vi "Main.vi"() -> ()   [LabVIEW 2010]
uses:
  <vilib>/Platform/storage/lvStorage.llb/xStorage/Open Data Storage/Open Data Storage.xnode
  <vilib>/Platform/storage/lvStorage.llb/xStorage/Set Properties/Set Properties.xnode
  <vilib>/Platform/storage/lvStorage.llb/xStorage/Write Data/Write Data.xnode
  <vilib>/Platform/storage/Storage.llb/usiOverwriteOptions.ctl
  <vilib>/Platform/storage/Storage.llb/usiSequenceRepresentation.ctl
  <vilib>/Platform/storage/lvStorage.llb/xStorage/Close Data Storage/Close Data Storage.xnode
  <instrlib>/Tektronix DPO MSO 2000 4000 Series/Public/Data/Read (Single Waveform).vi
  <instrlib>/Tektronix DPO MSO 2000 4000 Series/Public/Data/Read (Multiple Waveforms).vi
  <instrlib>/Tektronix DPO MSO 2000 4000 Series/Public/Configure/Configure Math (Dual).vi
  <vilib>/Platform/storage/lvStorage.llb/_openStorageWithRootAutoDetect.vi
  <vilib>/Platform/storage/lvStorage.llb/xStorage/xStorageSupp/ErrorOut.vi
  <vilib>/Platform/storage/Storage.llb/__savePropString.vi
  <vilib>/Platform/storage/Storage.llb/__savePropTime.vi
  <vilib>/Platform/storage/Storage.llb/_createExplicitChildObject.vi
  <vilib>/Platform/storage/lvStorage.llb/_prepDDT.vi
  <vilib>/Platform/storage/lvStorage.llb/_getChannelNameFromDDT.vi
  <vilib>/Platform/storage/lvStorage.llb/_saveDDT.vi
  <vilib>/Platform/storage/Storage.llb/Get Object Info.vi
  <vilib>/Platform/storage/Storage.llb/__closeStorageFromObject.vi
  <instrlib>/Tektronix DPO MSO 2000 4000 Series/Tektronix DPO MSO 2000 4000 Series.lvlib
panel:
  out "concatenated string":string
  out "Path 3":path
  out "error out":errorcluster
  out "down":bool
  out "up":bool
  out "DOWN":dbl
  out "UP":dbl
  in  "Error Range":dbl min=0.0 max=5.0 step=0.1 format="%#.3g"
  in  "Port to test":u16(ring) items=["AMB 1", "AMB 2", "AMB 3", "AMB 4", "AMB 5", "AMB 18"]
  in  "Assembled by":string="Alexis Ibarra"
  in  "ABM-S/N":string
  in  "IP Addres":string
  in  "Tab Control":T1(tab)
  in  "Start TEST":bool
  out "TIMA":waveform(dbl)(graph)
  out "TIMB":waveform(dbl)(graph)
  out "Differential Signal":waveform(dbl)(graph)
  out "TE Signals":waveform(dbl)[](graph)
  in  "Maximum Time (10000ms)":u32=20000
  in  "Channel B (1: Channel 2)":u16(ring)=1 items=["Channel 1", "Channel 2", "Channel 3", "Channel 4", "Math", "Reference 1", "Reference 2", "Reference 3", "Reference 4"]
  in  "Channel A (0: Channel 1)":u16(ring) items=["Channel 1", "Channel 2", "Channel 3", "Channel 4", "Math", "Reference 1", "Reference 2", "Reference 3", "Reference 4"]
  out "Periode":dbl
  out "Averenge":dbl
  out "STATUS":string
  # "ABM Verification System"
  # "%"
  # "Copyrigth Alexis Ibarrra A. ALMA  Computing"
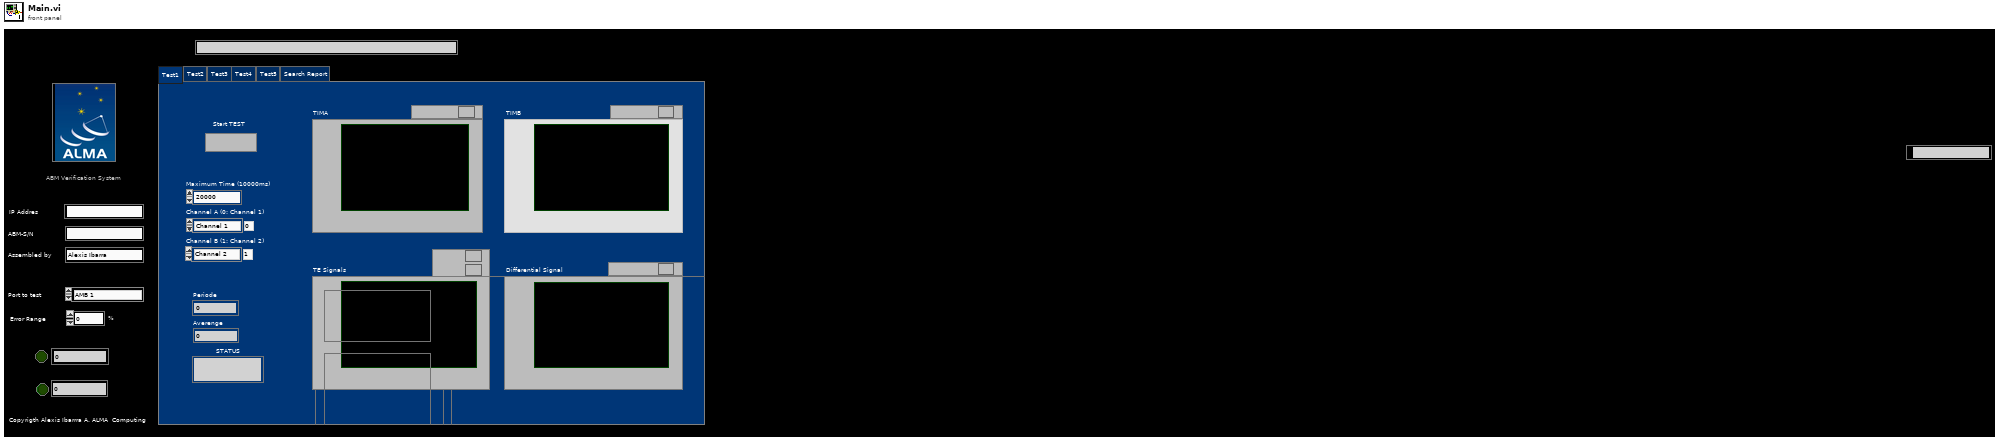
[diagram p1: front panel]
types:
  T1 = enum32{"Test1", "Test2", "Test3", "Test4", "Test5", "Search Report"}
  T2 = enum16{"open", "open or create", "create or replace", "create", "open (read only)"}
  T3 = enum16{"UPDATE", "READ", "QUERY", "CREATE CHILD", "CREATE", "CONNECT", "DISCONNECT"}
  T4 = typedef "usiOverwriteOptions.ctl" = enum16{"Append values", "Replace values at index", "Replace all values", "Append if timeline aligns"}
  T5 = typedef "usiSequenceRepresentation.ctl" = enum16{"explicit", "implicit"}
  T6 = enum32{"invalid app kind", "Development System", "Run Time System", "Student Edition", "Embedded LabVIEW", "Evaluation", "Custom"}
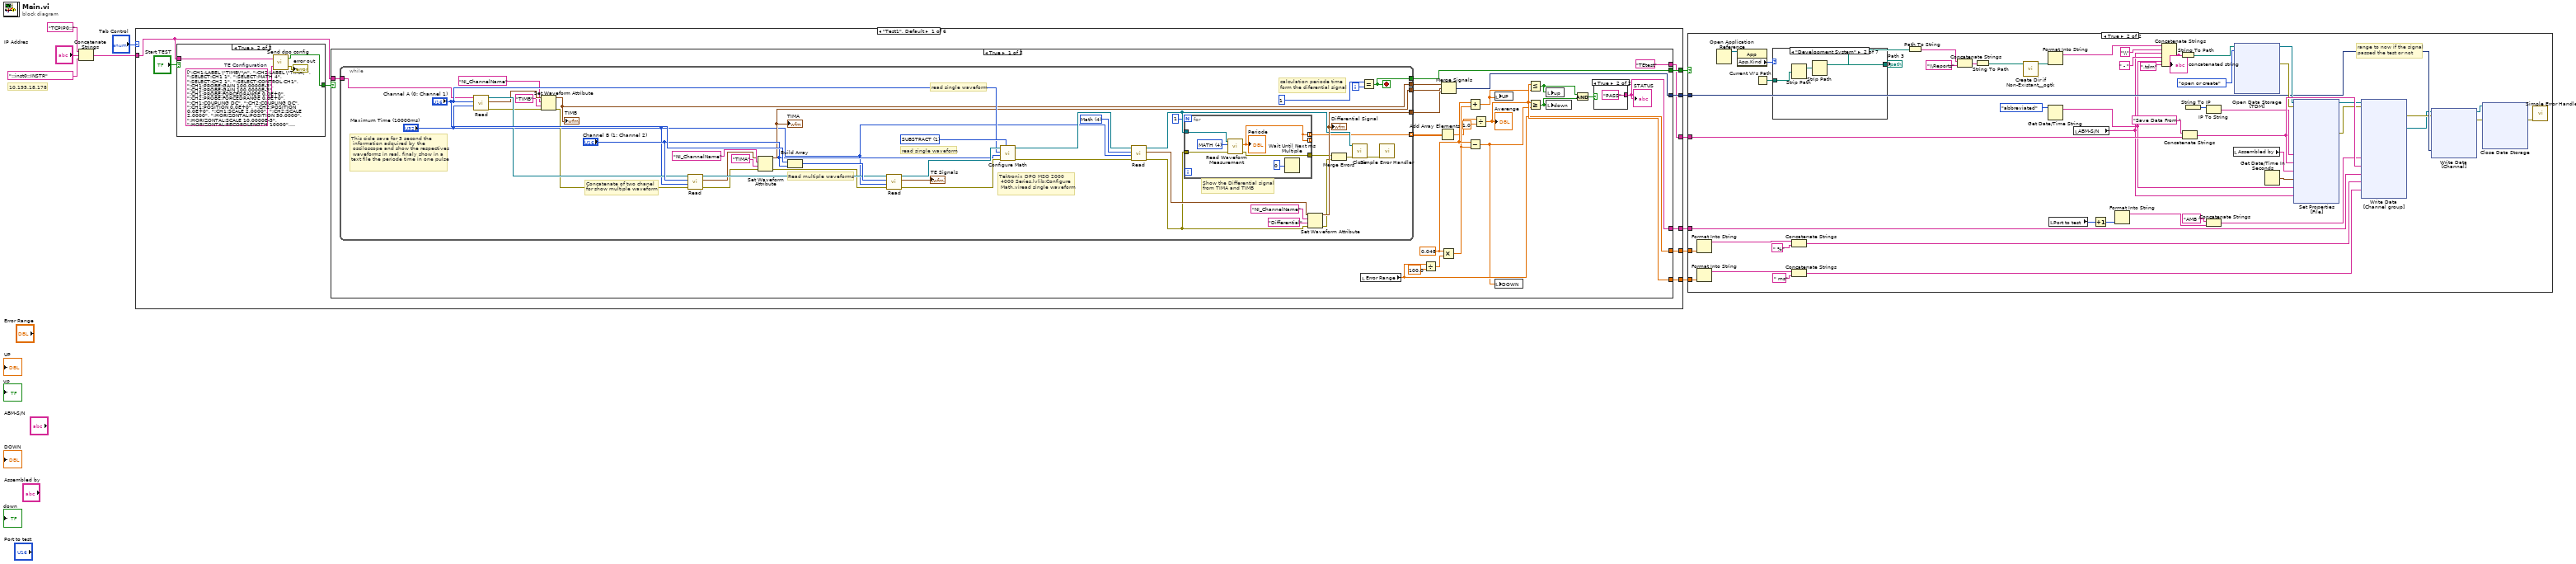
[diagram p0: block diagram]
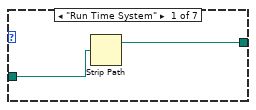
[diagram p3: hidden frame]
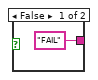
[diagram p9: hidden frame]
diagram:
  # "10.195.18.178"
  n1 = Concatenate Strings("TCPIP0::", "IP Addres", "::inst0::INSTR") -> (w7:string)
  n2 = case shown="\"Test1\", Default" "Tab Control" {
    tunnel: w7 -> [w18 _ _ _ _ _]
    tunnel: [w17 _ _ _ _ _] -> w6
    tunnel: [w16 _ _ _ _ _] -> w5
    tunnel: [w15 _ _ _ _ _] -> w4
    tunnel: [w14 _ _ _ _ _] -> w3
    tunnel: [w13 _ _ _ _ _] -> w2
    tunnel: [w12 _ _ _ _ _] -> w1
    frame "Test1", Default {
      n3 = case shown="True" "Start TEST" {
        tunnel: w18 -> [_ w94]
        tunnel: [_ w93] -> w19
        frame False {
        }
        frame True {
          w95 = string[] [":CH1:LABEL \"TIMB\"\n", ":CH2:LABEL \"TIMA\"", ":SELECT:CH1 1", ":SELECT:MATH 4", ":SELECT:CH2 1", ":SELECT:CONTROL CH1", ":CH1:PROBE:GAIN 100.0000E-3", ":CH2:PROBE:GAIN 100.0000E-3", ":CH1:PROBE:FORCEDRANGE 0.0E+0", ":CH2:PROBE:FORCEDRANGE 0.0E+0", ":CH1:COUPLING DC", ":CH2:COUPLING DC", ":CH1:POSITION 0.0E+0", ":CH2:POSITION 0.0E+0", ":CH1:SCALE 2.0000", ":CH2:SCALE 2.0000", ":HORIZONTAL:POSITION 50.0000", ":HORIZONTAL:SCALE 10.0000E-3", ":HORIZONTAL:RECORDLENGTH 10000", ":HORIZONTAL:DELAY:MODE 1", ":HORIZONTAL:DELAY:TIME 0.0E+0", ":TRIGGER:A:MODE AUTO", ":TRIGGER:A:TYPE EDGE", ":TRIGGER:A:LEVEL 2.0000", ":TRIGGER:A:LEVEL:CH2 2.0000", ":TRIGGER:A:UPPERTHRESHOLD:CH2 2.2000", ":TRIGGER:A:LOWERTHRESHOLD:CH2 2.000", ":TRIGGER:A:HOLDOFF:TIME 20.0000E-9", ":TRIGGER:A:EDGE:SOURCE CH2", ":TRIGGER:A:EDGE:COUPLING DC", ":TRIGGER:A:LOGIC:THRESHOLD:CH2 2.0000", ":TRIGGER:A:SETHOLD:DATA:SOURCE CH2", ":TRIGGER:A:SETHOLD:DATA:THRESHOLD 2.0000", ":ZOOM:GRATICULE:SIZE 80", ":DATA:SOURCE CH2", ":MATH:POSITION -3.00E-3", ":MATH:SCALE 2.0000"]  # TE Configuration
          n4 = call "Send dpo config.vi"("Array Configuration"=w95, "TCP/IP Addres"=w94) -> ("error out"=→"error out":errorcluster, "Exit"=w93:bool)
        }
      }
      n5 = case shown="True" w19 {
        tunnel: w18 -> [w42 _]
        tunnel: [w30 _] -> w17
        tunnel: [w29 _] -> w16
        tunnel: [w28 _] -> w15
        tunnel: [w27 _] -> w14
        tunnel: [w26 _] -> w13
        tunnel: ["TEtest" _] -> w12
        frame True {
          w39 = 0.048 ("x")
          n6 = while {
            tunnel: [w57] -> w36
            tunnel: w42 -> [w72]
            tunnel: [w69] -> w34
            tunnel: [w61] -> w35
            tunnel: [w43] -> w30
            tunnel: [w45] -> w33 mode=indexing
            i -> [w47]
            stop <- w43 stop-if-true
            w53 = u16 4 items=["Channel 1", "Channel 2", "Channel 3", "Channel 4", "Math", "Reference 1", "Reference 2", "Reference 3", "Reference 4"] ("Channel (0: Channel 1)")
            w80 = u16 1 items=["ADD", "SUBSTRACT", "MULTIPLY", "DIVIDE"] ("Operator (0: ADD)")
            # "This cicle save for 3 second the\n information adquired by the\n osciloscope and show the respectives\n waveforms in real, finaly show in a \ntext file the periode time in one pulse"
            # "Concatenate of two chanel \nfor show multiple waveform"
            # "read single waveform"
            # "read single waveform"
            # "Tektronix DPO MSO 2000\n 4000 Series.lvlib:Configure\n Math.viread single waveform"
            # "calculation periode time\nform the diferential signal"
            # "Show the Differential signal \nfrom TIMA and TIMB"
            # "Read multiple waveforms"
            n7 = call-poly <instrlib>:"Read.vi"("Maximum Time (10000ms)"="Maximum Time (10000ms)", "Channel (0: Channel 1)"="Channel A (0: Channel 1)", "VISA resource name"=w72) -> ("error out"=w68:errorcluster, "Waveform Graph"=w71:waveform(dbl), "VISA resource name out"=w74:refnum<visa-resource-name>)  [unwired: 6 in]
            n8 = Set Waveform Attribute(4:w68, 5:"TIMB" ("name"), 6:"NI_ChannelName" ("name"), 7:w71) -> (0:w67:errorcluster, 3:w69:waveform(dbl))  [unwired: 1 out]
            "TIMB" <- w69
            n9 = call-poly <instrlib>:"Read.vi"("error in (no error)"=w67, "Maximum Time (10000ms)"="Maximum Time (10000ms)", "Channel (0: Channel 1)"="Channel B (1: Channel 2)", "VISA resource name"=w74) -> ("error out"=w63:errorcluster, "Waveform Graph"=w64:waveform(dbl), "VISA resource name out"=w73:refnum<visa-resource-name>)  [unwired: 5 in]
            n10 = Set Waveform Attribute(4:w63, 5:"TIMA" ("name"), 6:"NI_ChannelName" ("name"), 7:w64) -> (0:w62:errorcluster, 3:w61:waveform(dbl))  [unwired: 1 out]
            "TIMA" <- w61
            n11 = Build Array("Channel A (0: Channel 1)", "Channel B (1: Channel 2)") -> (w82:u16[])
            n12 = call-poly <instrlib>:"Read.vi"("error in (no error)"=w62, "Maximum Time (10000ms)"="Maximum Time (10000ms)", "Channels"=w82, "VISA resource name"=w73) -> ("error out"=w81:errorcluster, "Waveform Data"=→"TE Signals":waveform(dbl)[], "VISA resource name out"=w78:refnum<visa-resource-name>)  [unwired: 5 in]
            n13 = call-poly <instrlib>:"Configure Math.vi"("Operator (0: ADD)"=w80, "error in (no error)"=w81, "2nd Source (1: Channel 2)"="Channel B (1: Channel 2)", "1st Source (0: Channel 1)"="Channel A (0: Channel 1)", "VISA resource name"=w78) -> ("error out"=w77:errorcluster, "VISA resource name out"=w79:refnum<visa-resource-name>)  [unwired: 5 in]
            n14 = call-poly <instrlib>:"Read.vi"("error in (no error)"=w77, "Maximum Time (10000ms)"="Maximum Time (10000ms)", "Channel (0: Channel 1)"=w53, "VISA resource name"=w79) -> ("error out"=w51:errorcluster, "Waveform Graph"=w58:waveform(dbl), "VISA resource name out"=w52:refnum<visa-resource-name>)  [unwired: 5 in]
            n15 = for {
              N: 1 -> [_]
              tunnel: w52 -> [w89]
              tunnel: w51 -> [w87]
              tunnel: [w85] -> w50
              tunnel: [w84] -> _ mode=indexing
              tunnel: [w84] -> w45 mode=indexing
              w88 = u16 4 items=["Channel 1", "Channel 2", "Channel 3", "Channel 4", "MATH", "Reference 1", "Reference 2", "Reference 3", "Reference 4"] ("Channel (0: Channel 1)")
              n16 = call <instrlib>:"Read Waveform Measurement.vi"("error in (no error)"=w87, "Channel (0: Channel 1)"=w88, "VISA resource name"=w89) -> ("error out"=w85:errorcluster, "Measurement Value"=w84:dbl)  [unwired: 6 in, 1 out]
              "Periode" <- w84
              n17 = Wait Until Next ms Multiple(millisecond multiple=u32 0) -> ()  [unwired: 1 out]
            }
            n18 = Set Waveform Attribute(4:w51, 5:"Differential" ("name"), 6:"NI_ChannelName" ("name"), 7:w58) -> (0:w49:errorcluster, 3:w57:waveform(dbl))  [unwired: 1 out]
            "Differential Signal" <- w57
            n19 = Merge Errors(w50, w49) -> (w48:errorcluster)
            n20 = call <instrlib>:"Close.vi"("error in (no error)"=w48, "VISA resource name"=w52) -> ("error out"=w83:errorcluster)  [unwired: 9 in]
            n21 = Equal?(x=1, y=w47) -> (x = y?=w43:bool)
            n22 = call <vilib>:"Simple Error Handler.vi"("error in (no error)"=w83) -> ()  [unwired: 4 in, 5 out]
          }
          n23 = local read "Error Range"() -> (w26:dbl)
          n24 = Divide(x=w26, y=100.0) -> (x/y=w40:dbl)
          n25 = Add Array Elements(numeric array=w33) -> (sum=w32:dbl)
          n26 = Multiply(x=w39, y=w40) -> (x*y=w38:dbl)
          n27 = Merge Signals "Merge Signals"(w34, w35, w36) -> (w29:dynamicdata)
          n28 = Add(x=w39, y=w38) -> (x+y=w25:dbl)
          n29 = Subtract(x=w39, y=w38) -> (x-y=w24:dbl)
          n30 = Divide(x=w32, y=1.0) -> (x/y=w27:dbl)
          "Averenge" <- w27
          n31 = local write "UP"(w25) -> ()
          n32 = local write "DOWN"(w24) -> ()
          n33 = Less Or Equal?(x=w27, y=w25) -> (x <= y?=w23:bool)
          n34 = Greater Or Equal?(x=w27, y=w24) -> (x >= y?=w22:bool)
          n35 = local write "up"(w23) -> ()
          n36 = local write "down"(w22) -> ()
          n37 = And(x=w23, y=w22) -> (x .and. y?=w37:bool)
          n38 = case shown="True" w37 {
            tunnel: ["FAIL" "PASS"] -> w28
            frame False {
            }
            frame True {
            }
          }
          "STATUS" <- w28
        }
        frame False {
        }
      }
    }
    frame "Test2" {
    }
    frame "Test3" {
    }
    frame "Test4" {
    }
    frame "Test5" {
    }
    frame "Search Report" {
    }
  }
  n39 = case shown="True" w6 {
    tunnel: w3 -> [_ w126]
    tunnel: w2 -> [_ w125]
    tunnel: w4 -> [_ w124]
    tunnel: w5 -> [_ w120]
    tunnel: w1 -> [_ w121]
    frame False {
    }
    frame True {
      # "range to now if the signal\npassed the test or not"
      n40 = Format Into String "Format Into String"(w125) -> (resulting string=w136:string)  [unwired: 3 in, 1 out]
      n41 = Format Into String "Format Into String"(w126) -> (resulting string=w134:string)  [unwired: 3 in, 1 out]
      n42 = Open Application Reference() -> (3:w107:refnum<vi>)  [unwired: 4 in, 1 out]
      n43 = property class="App"(reference=w107) -> ("App.Kind"=w106:T6)  [unwired: 1 in, 2 out]
      n44 = Current VI's Path() -> (path=w105:path)
      n45 = case shown="\"Development System\"" w106 {
        tunnel: w105 -> [w147 w149 _ _ _ _ _]
        tunnel: [w146 w148 _ _ _ _ _] -> w104
        frame "Run Time System" {
          n46 = Strip Path(path=w147) -> (stripped path=w146:path)  [unwired: 1 out]
        }
        frame "Development System" {
          n47 = Strip Path(path=w149) -> (stripped path=w150:path)  [unwired: 1 out]
          n48 = Strip Path(path=w150) -> (stripped path=w148:path)  [unwired: 1 out]
        }
        frame "Student Edition" {
        }
        frame "Embedded LabVIEW" {
        }
        frame "Evaluation" {
        }
        frame "Custom" {
        }
        frame "invalid app kind" {
        }
      }
      "Path 3" <- w104
      n49 = Concatenate Strings "Concatenate Strings"(w136, " %") -> (w143:string)
      n50 = Concatenate Strings "Concatenate Strings"(w134, " ms") -> (w144:string)
      n51 = Path To String(path=w104) -> (string=w103:string)
      n52 = Concatenate Strings(w103, "\\Reports") -> (w100:string)
      n53 = String To Path(string=w100) -> (path=w101:path)
      n54 = call <userlib>:"Create Dir if Non-Existant__ogtk.vi"("Directory Path"=w101) -> ("dup Directory Path"=w99:path)  [unwired: 8 in, 2 out]
      n55 = Format Into String "Format Into String"(w99) -> (resulting string=w97:string)  [unwired: 3 in, 1 out]
      n56 = Get Date/Time String(date format (0)=enum16{"short", "long", "abbreviated"}."abbreviated") -> (date string=w108:string)  [unwired: 2 in, 1 out]
      n57 = local read "Port to test"() -> (w123:u16)
      n58 = local read "ABM-S/N"() -> (w110:string)
      n59 = Increment(x=w123) -> (x+1=w133:u16)
      n60 = Format Into String "Format Into String"(w133) -> (resulting string=w139:string)  [unwired: 3 in, 1 out]
      n61 = Concatenate Strings(w97, "\\" ("string"), w110, " - ", w108, ".tdm") -> (w98:string)
      "concatenated string" <- w98
      n62 = String To Path(string=w98) -> (path=w109:path)
      n63 = Concatenate Strings "Concatenate Strings"("Save Data From ", w121) -> (w145:string)
      n64 = String To IP() -> (0:w132:u32)  [unwired: 1 in]
      n65 = IP To String(2:w132) -> (0:w131:string)  [unwired: 1 in]
      n66 = Concatenate Strings "Concatenate Strings"("AMB ", w139) -> (w142:string)
      n67 = local read "Assembled by"() -> (w122:string)
      n68 = xnode "Open Data Storage\n[TDM]"("file path"=w109, "function (open:0)"=T2."open or create") -> ("storage refnum (file)"=w129:refnum<k20>, "error out"=w138:errorcluster)  [unwired: 3 in, 1 out]
      n69 = Get Date/Time In Seconds() -> (seconds since 1Jan1904=w128:timestamp)
      n70 = xnode "Set Properties\n[File]"("Name"=w131, "Description"=w145, "Author"=w122, "Time stamp"=w128, "Date"=w108, "ABM_SerialNumber"=w110, "storage refnum (file)"=w129, "error in"=w138) -> ("storage refnum (file) out"=w140:refnum<k20>, "error out"=w141:errorcluster)
      n71 = xnode "Write Data\n[Channel group]"("storage refnum (file)"=w140, "error in"=w141, "Name"=w142, "Description"=w145, "Status"=w124, "Error_Range"=w143, "Periode"=w144) -> ("error out"=w119:errorcluster, "storage refnum (channel group)"=w118:refnum<k20>)  [unwired: 1 out]
      n72 = xnode "Write Data\n[Channel]"("Signal"=w120, "storage refnum (channel group)"=w118, "error in"=w119) -> ("storage refnum (channel group) out"=w116:refnum<k20>, "error out"=w115:errorcluster)  [unwired: 2 in, 1 out]
      n73 = xnode "Close Data Storage\n"("storage refnum (channel group)"=w116, "error in (no error)"=w115) -> ("error out"=w117:errorcluster)  [unwired: 1 out]
      n74 = call <vilib>:"Simple Error Handler.vi"("error in (no error)"=w117) -> ()  [unwired: 1 in, 8 out]
    }
  }
